vi "Calculate FFT Length From Record Length.vi"(8 "error in (no error)":errorcluster, 11 "Record Length In":u32=1536) -> (0 "error out":errorcluster, 2 "FFT Length":u32, 3 "Record Length Out":u32=1536)   [LabVIEW 2018]
panel:
  out "Array":u32[](array[numeric])
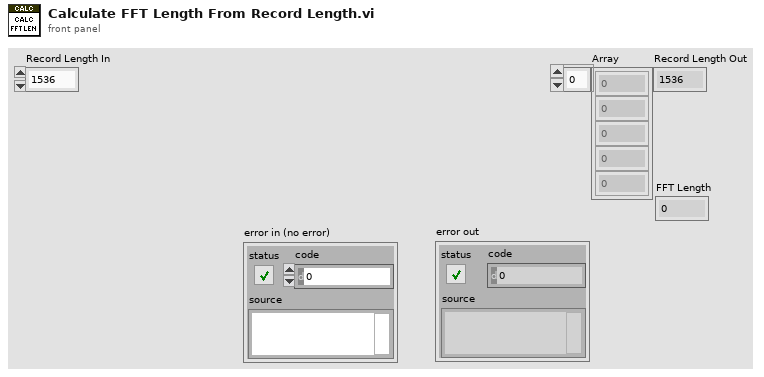
[diagram p1: front panel]
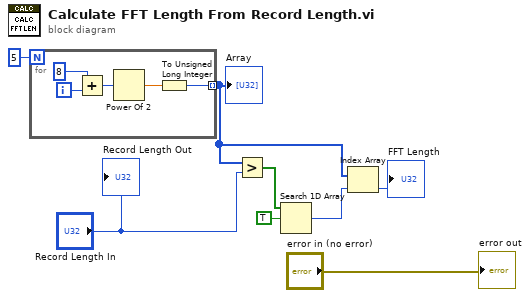
[diagram p0: block diagram]
diagram:
  n1 = for {
    N: 5 -> [_]
    tunnel: [w9] -> w4 mode=indexing
    i -> [w13]
    n2 = Add(x=8, y=w13) -> (x+y=w12:i32)
    n3 = Power Of 2(x=w12) -> (2^x=w10:dbl)
    n4 = To Unsigned Long Integer(number=w10) -> (unsigned 32bit integer=w9:u32)
  }
  "Array" <- w4
  n5 = Greater?(x=w4, y="Record Length In") -> (0:w7:bool[])
  n6 = Search 1D Array(1D array=w7, element=TRUE) -> (index of element=w5:i32)  [unwired: 1 in]
  n7 = Index Array(array=w4, index=w5) -> (element=→"FFT Length":u32)
  "error out" <- "error in (no error)"
  "Record Length Out" <- "Record Length In"
